vi "Trapezoidal Acceleration.vi"(8 "AccelRate":dbl, 9 "Desired":dbl, 10 "Actual":dbl, 11 "LoopTime":dbl) -> (2 "New Actual":dbl)   [LabVIEW 2013]
doc: "Fixes motor acceleration to a linear rate."
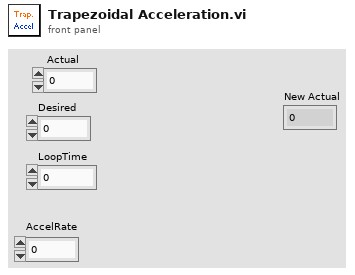
[diagram p1: front panel]
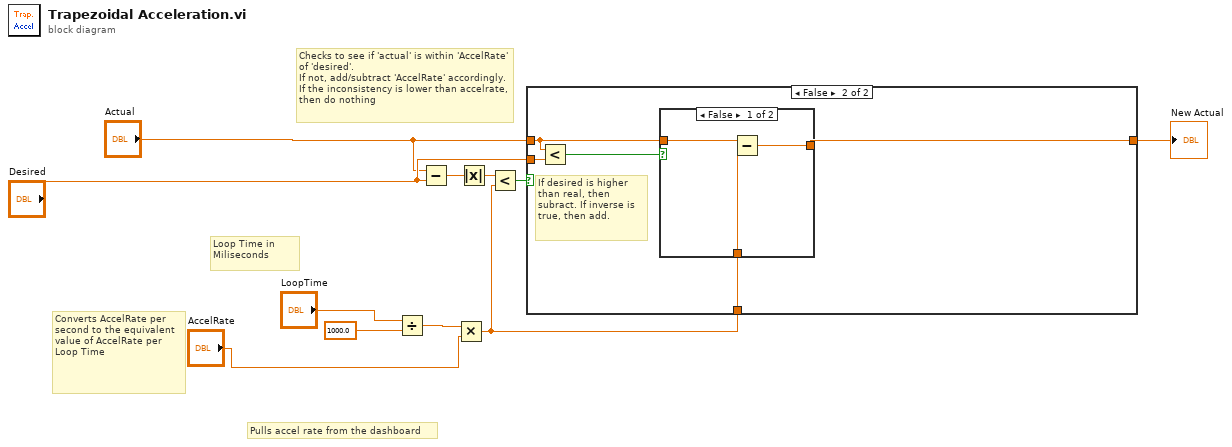
[diagram p0: block diagram]
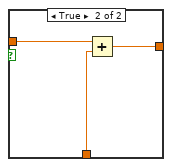
[diagram p3: hidden frame]
diagram:
  # "Pulls accel rate from the dashboard"
  # "Checks to see if 'actual' is within 'AccelRate' of 'desired'.\nIf not, add/subtract 'AccelRate' accordingly. If the inconsistency is lower than accelrate, then do nothing"
  # "Converts AccelRate per second to the equivalent value of AccelRate per Loop Time"
  # "Loop Time in Miliseconds"
  n1 = Divide(x="LoopTime", y=1000.0) -> (x/y=w7:dbl)
  n2 = Subtract(x="Actual", y="Desired") -> (x-y=w10:dbl)
  n3 = Multiply(x=w7, y="AccelRate") -> (x*y=w6:dbl)
  n4 = Absolute Value(x=w10) -> (abs(x)=w11:dbl)
  n5 = Less?(x=w11, y=w6) -> (x < y?=w9:bool)
  n6 = case shown="False" w9 {
    tunnel: [w12 w17] -> w5
    tunnel: "Actual" -> [w12 w16]
    tunnel: "Desired" -> [_ w14]
    tunnel: w6 -> [_ w13]
    frame True {
    }
    frame False {
      # "If desired is higher than real, then subract. If inverse is true, then add."
      n7 = Less?(x=w16, y=w14) -> (x < y?=w15:bool)
      n8 = case shown="False" w15 {
        tunnel: w16 -> [w18 w22]
        tunnel: [w20 w23] -> w17
        tunnel: w13 -> [w19 w21]
        frame False {
          n9 = Subtract(x=w18, y=w19) -> (x-y=w20:dbl)
        }
        frame True {
          n10 = Add(x=w22, y=w21) -> (x+y=w23:dbl)
        }
      }
    }
  }
  "New Actual" <- w5
